vi "state_machine.vi"(4 "Extension Pos Actual":dbl, 5 "Rotation Pos Actual":dbl, 10 "ArmData":T1) -> (0 "ExtensionDesired":dbl, 2 "Rotation Rate":dbl=1.0, 3 "RotationDesired":dbl, 6 "Current_State":string)   [LabVIEW 2011]
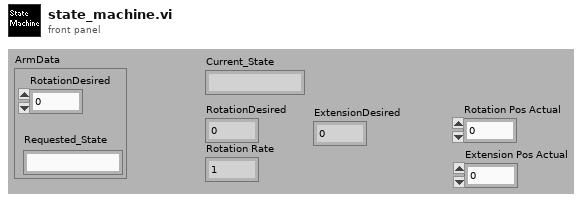
[diagram p1: front panel]
types:
  T1 = cluster{"RotationDesired":dbl, "Requested_State":string}
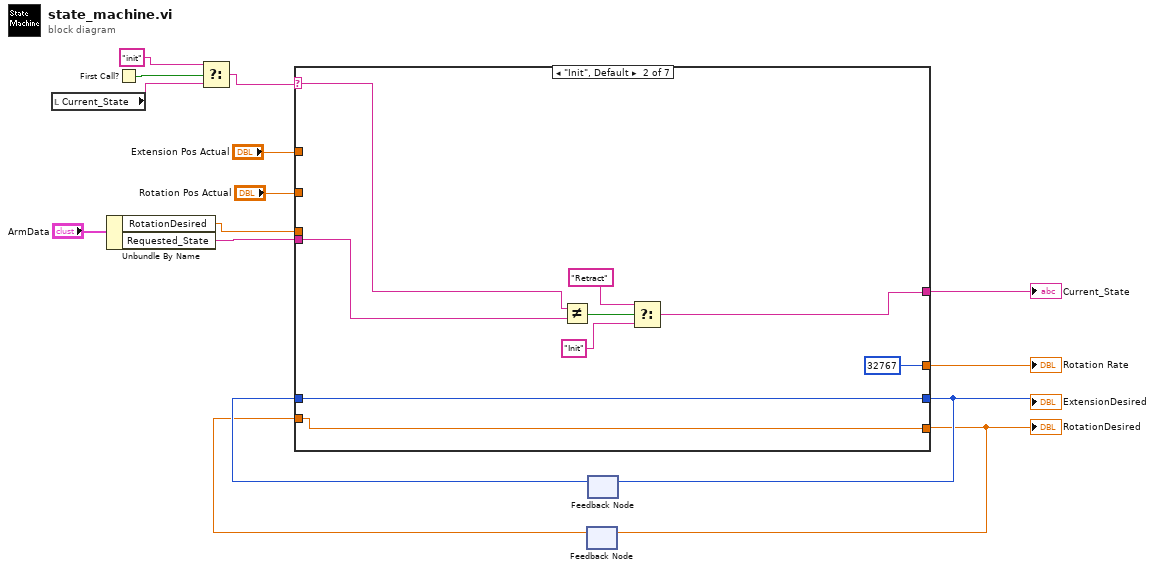
[diagram p0: block diagram]
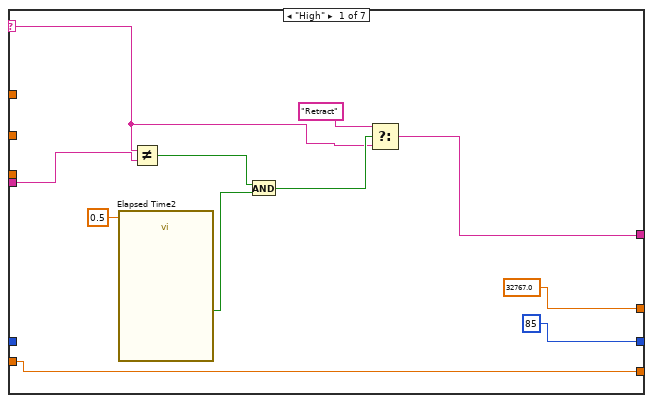
[diagram p2: hidden frame]
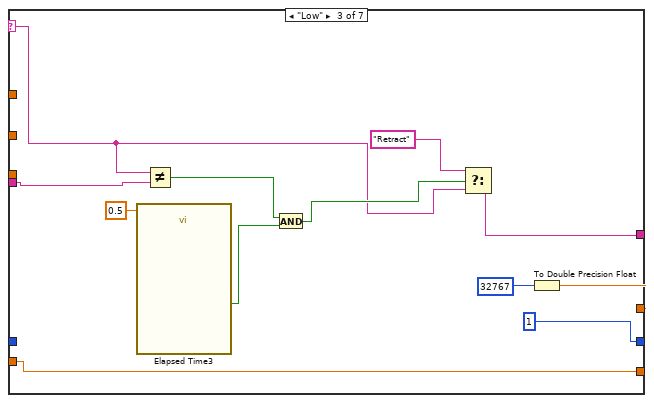
[diagram p3: hidden frame]
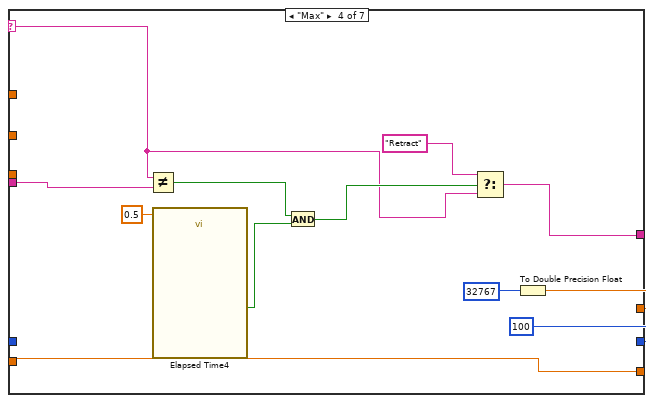
[diagram p4: hidden frame]
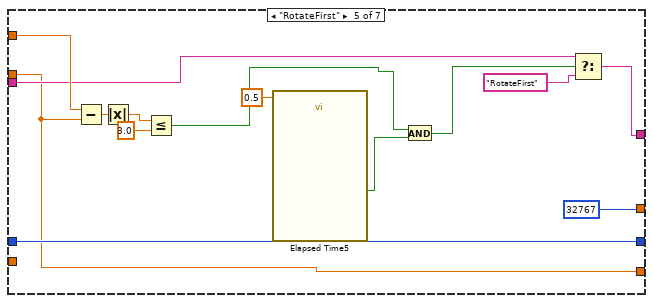
[diagram p5: hidden frame]
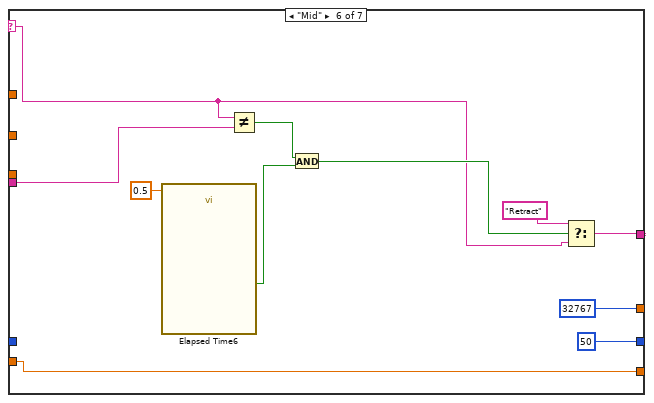
[diagram p6: hidden frame]
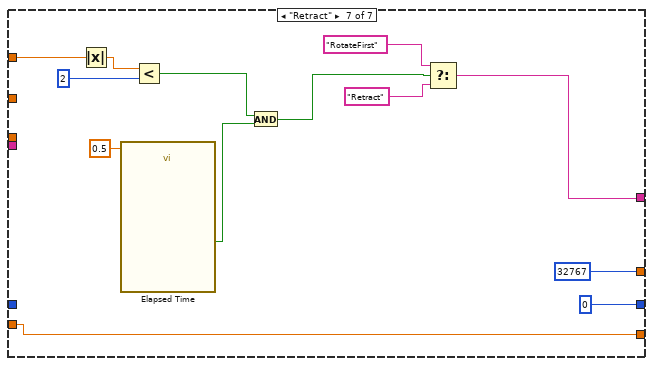
[diagram p7: hidden frame]
diagram:
  n1 = local read "Current_State"() -> (w1:string)
  n2 = Unbundle By Name("ArmData") -> ("RotationDesired"=w8:dbl, "Requested_State"=w7:string)
  n3 = First Call?() -> (First Call?: T/F=w4:bool)
  n4 = Select(t="init", s=w4, f=w1) -> (s? t:f=w2:string)
  n5 = feedback #1() -> (w5:dbl)  [unwired: 1 out]
  n6 = feedback #2() -> (w14:i32)  [unwired: 1 out]
  n7 = case shown="\"Init\", Default" w2 {
    selector: w2 -> [w18 w31 w38 w49 _ w76 _]
    tunnel: [w26 w27 w45 w57 w72 w81 w86] -> w12
    tunnel: "Extension Pos Actual" -> [_ _ _ _ _ _ w92]
    tunnel: w7 -> [w19 w32 w39 w50 w65 w80 _]
    tunnel: [85 w34 1 100 w71 50 0] -> w10
    tunnel: [w16 w33 w36 w48 w64 w74 w90] -> w6
    tunnel: w14 -> [_ w34 _ _ w71 _ _]
    tunnel: "Rotation Pos Actual" -> [_ _ _ _ w68 _ _]
    tunnel: [32767.0 32767 w44 w56 32767 32767 32767] -> w11
    tunnel: w8 -> [_ _ _ _ w64 _ _]
    tunnel: w5 -> [w16 w33 w36 w48 _ w74 w90]
    frame "High" {
      n8 = call "Elapsed Time2"("Time Target (s)"=0.5) -> ("Time has Elapsed"=w22:bool)  [unwired: 4 in, 14 out]
      n9 = Not Equal?(x=w18, y=w19) -> (x != y?=w21:bool)
      n10 = And(x=w21, y=w22) -> (x .and. y?=w20:bool)
      n11 = Select(t="Retract", s=w20, f=w18) -> (s? t:f=w26:string)
    }
    frame "Init", Default {
      n12 = Not Equal?(x=w31, y=w32) -> (x != y?=w30:bool)
      n13 = Select(t="Retract", s=w30, f="Init") -> (s? t:f=w27:string)
    }
    frame "Low" {
      n14 = call "Elapsed Time3"("Time Target (s)"=0.5) -> ("Time has Elapsed"=w42:bool)  [unwired: 4 in, 14 out]
      n15 = Not Equal?(x=w38, y=w39) -> (x != y?=w41:bool)
      n16 = And(x=w41, y=w42) -> (x .and. y?=w40:bool)
      n17 = Select(t="Retract", s=w40, f=w38) -> (s? t:f=w45:string)
      n18 = To Double Precision Float(number=32767) -> (double precision float=w44:dbl)
    }
    frame "Max" {
      n19 = Not Equal?(x=w49, y=w50) -> (x != y?=w53:bool)
      n20 = call "Elapsed Time4"("Time Target (s)"=0.5) -> ("Time has Elapsed"=w54:bool)  [unwired: 4 in, 14 out]
      n21 = And(x=w53, y=w54) -> (x .and. y?=w52:bool)
      n22 = Select(t="Retract", s=w52, f=w49) -> (s? t:f=w57:string)
      n23 = To Double Precision Float(number=32767) -> (double precision float=w56:dbl)
    }
    frame "RotateFirst" {
      n24 = Subtract(x=w68, y=w64) -> (x-y=w67:dbl)
      n25 = Absolute Value(x=w67) -> (abs(x)=w66:dbl)
      n26 = Less Or Equal?(x=w66, y=3.0) -> (x <= y?=w62:bool)
      n27 = call "Elapsed Time5"("Time Target (s)"=0.5) -> ("Time has Elapsed"=w63:bool)  [unwired: 4 in, 14 out]
      n28 = And(x=w62, y=w63) -> (x .and. y?=w61:bool)
      n29 = Select(t=w65, s=w61, f="RotateFirst") -> (s? t:f=w72:string)
    }
    frame "Mid" {
      n30 = call "Elapsed Time6"("Time Target (s)"=0.5) -> ("Time has Elapsed"=w79:bool)  [unwired: 4 in, 14 out]
      n31 = Not Equal?(x=w76, y=w80) -> (x != y?=w78:bool)
      n32 = And(x=w78, y=w79) -> (x .and. y?=w77:bool)
      n33 = Select(t="Retract", s=w77, f=w76) -> (s? t:f=w81:string)
    }
    frame "Retract" {
      n34 = Absolute Value(x=w92) -> (abs(x)=w94:dbl)
      n35 = call "Elapsed Time"("Time Target (s)"=0.5) -> ("Time has Elapsed"=w89:bool)  [unwired: 4 in, 14 out]
      n36 = Less?(x=w94, y=2) -> (x < y?=w88:bool)
      n37 = And(x=w88, y=w89) -> (x .and. y?=w87:bool)
      n38 = Select(t="RotateFirst", s=w87, f="Retract") -> (s? t:f=w86:string)
    }
  }
  "Current_State" <- w12
  "ExtensionDesired" <- w10
  "RotationDesired" <- w6
  "Rotation Rate" <- w11
  n39 = feedback-in #1(w6) -> ()
  n40 = feedback-in #2(w10) -> ()
